vi "Beam_Max_Pos.vi"(1 "Picture Log":path, 5 "Search Step (mm)":dbl=1.0, 6 "Mode":T6, 7 "Starting Position":dbl[](array[numeric]) format="%.1f", 8 "Traverse line In":T1 {"Row Duration (mins)" format="%#.1f"; "Row No" min=0; "Trace Gas Concentration (%)" min=0.0 format="%#.2f"; "Emission Rate (l/min)" format="%#.2f"; "Tunnel Speed" format="%#.2f"; "Start X" format="%#.2f"; "Start Y" format="%#.2f"; "Start Z" format="%#.2f"; "End X" format="%#.2f"; "End Y" format="%#.2f"; "End Z" format="%#.2f"; "Averaging time (min)" min=0.0 format="%#.2f"}, 9 "Fixed Axis":T4, 10 "Beam Name":string) -> (0 "Power at Maxima":dbl, 2 "Status":T5, 3 "Beam maxima":dbl[](array[numeric]) format="%.1f", 4 "Message":string)   [LabVIEW 2010]
uses:
  Controls/User_Specific_mode.ctl
  Gen Trav/Multi_Run_Status.ctl
  Gen Trav/Route mapping/Axis.ctl
  Gen Trav/Traverse_cluster.ctl
  Gen Trav/Spacing.ctl
  Controls/Multi_run_mode.ctl
  File/Setup_Filetype.ctl
panel:
  out "Server copy Location":path
  out "vi reference":refnum<vi>
  in  "stop":bool
  out "Y":i32
  out "X":i32
  out "Array 2":dbl[](array[numeric]) format="%.4f"
  out "Measured Points":dbl[][](array[numeric]) format="%.2f"
  out "Current Value":dbl format="%.2f"
  out "Current Index":i32
  out "Array":i32[][](array[numeric])
  out "Light Power Measurement":dbl[][](graph)
  out "Found Maxima?":bool
  out "Present Position":dbl[](array[numeric])
  out "Profile":dbl[][](array[numeric]) format="%.2f"
  out "Log File":path
  # "X           Y            Z"
  # "Start"
  # "End"
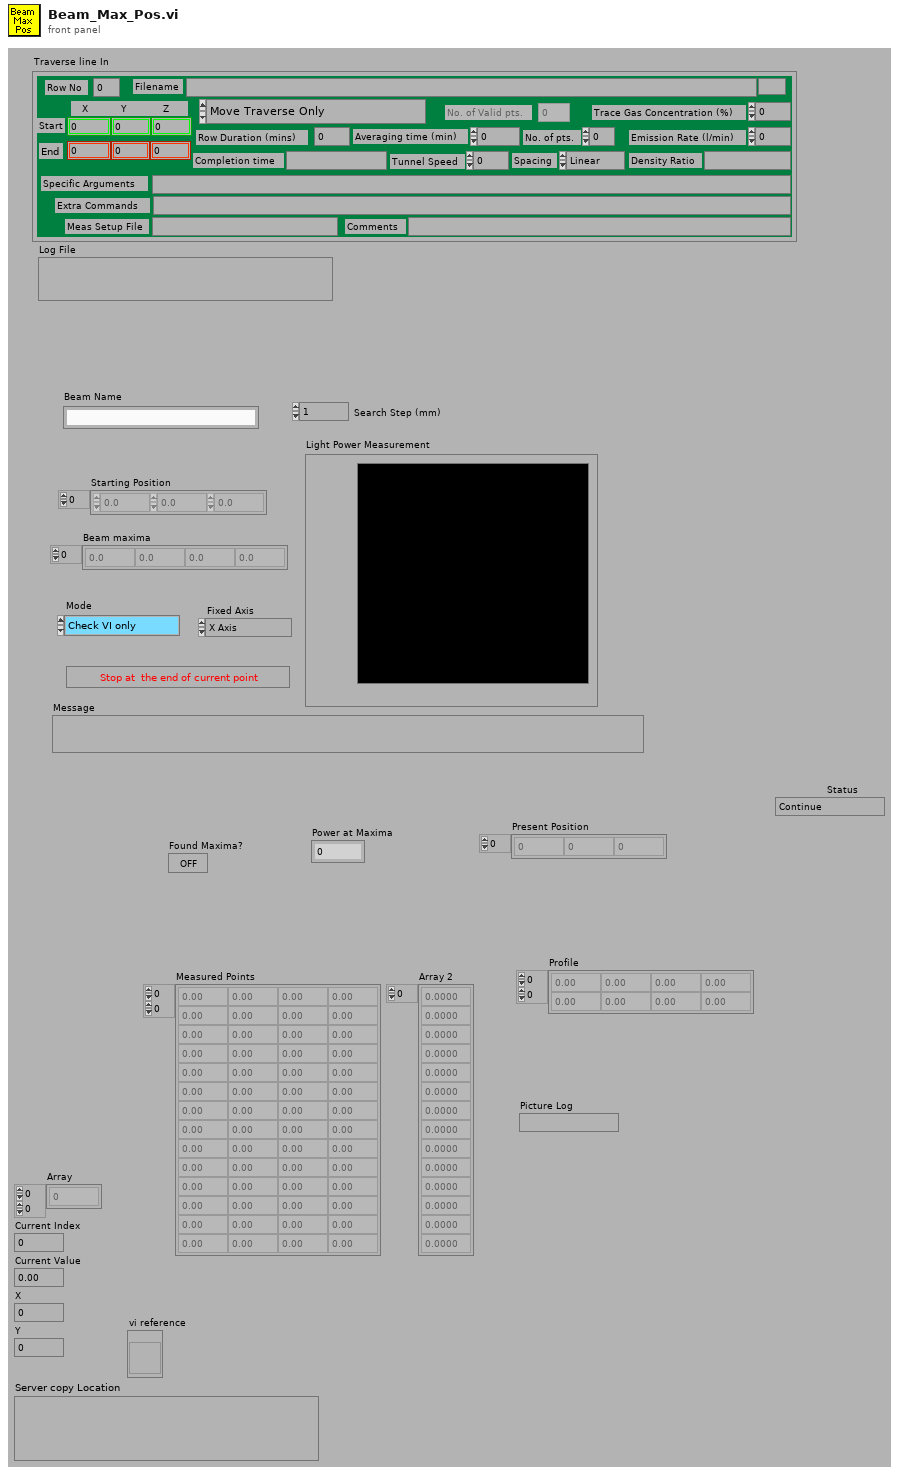
[diagram p1: front panel]
types:
  T1 = typedef "Traverse_cluster.ctl" = cluster{"Start X":dbl, "Start Y":dbl, "Start Z":dbl, "End X":dbl, "End Y":dbl, "End Z":dbl, "No. of pts.":i32, "Spacing":T2, "Filename":path, "Tunnel Speed":dbl, "Averaging time (min)":dbl, "Extra Commands":string, "Specific Arguments":string, "Emission Rate (l/min)":dbl, "Trace Gas Concentration (%)":dbl, "Density Ratio":string, "Comments":string, "Row No":i32, "Row Type Selector":T3, "Completion time":string, "Row Duration (mins)":dbl, "No. of Valid pts.":i32, "Meas Setup File":string}
  T2 = typedef "Spacing.ctl" = enum16{"Linear", "Log", "Gauss", "Specified", "N/A"}
  T3 = typedef "Multi_run_mode.ctl" = enum16{"Move Traverse Only", "Set Tunnel Speed Only", "Set Source Only", "Set Measurement Conditions", "Single Measurement", "Vertical Profile", "Lateral Profile", "Longitudinal Profile", "Explore Volume", "Multi-Axis Profile", "Auto Calibrate", "Meas Fast FID Bkgnd", "Check Beam Power", "Scanning Valve Measurement", "Run VI Named:", "Set ADAM Ch", "Wait (minutes)", "Send Message", "Synchronize With:", "Fall Back to this Row", "Turn Off Row Repeating", "Blank Row"}
  T4 = typedef "Axis.ctl" = enum16{"X Axis", "X Axis -ve", "Y Axis", "Y Axis -ve", "Z Axis", "Z Axis -ve"}
  T5 = typedef "Multi_Run_Status.ctl" = enum16{"Continue", "Jump to Next Point", "Jump to Next Row", "Jump To Fall Back", "Terminate Run"}
  T6 = typedef "User_Specific_mode.ctl" = enum16{"Check VI only", "Run VI"}
  T7 = typedef "Setup_Filetype.ctl" = enum16{"Measurement Setups", "Calibration Setups", "General", "Results File Plotter Setups", "Speed Calib Tweaks"}
  T8 = cluster{"Status":enum16{"Continue", "Jump to Next Point", "Jump to Next Row", "Jump To Fall Back", "Terminate Run"}, "Error Type":string, "Error Description":string}
  T9 = typedef "Status_Cluster.ctl" = cluster{"Status":T5, "Error Type":string, "Error Description":string}
  T10 = cluster{"second":i32, "minute":i32, "hour":i32, "day of month":i32, "month":i32, "year":i32, "day of week":i32, "day of year":i32, "is DST":i32}
  T11 = typedef "LVRectTypeDef.ctl" = cluster{"left":i16, "top":i16, "right":i16, "bottom":i16}
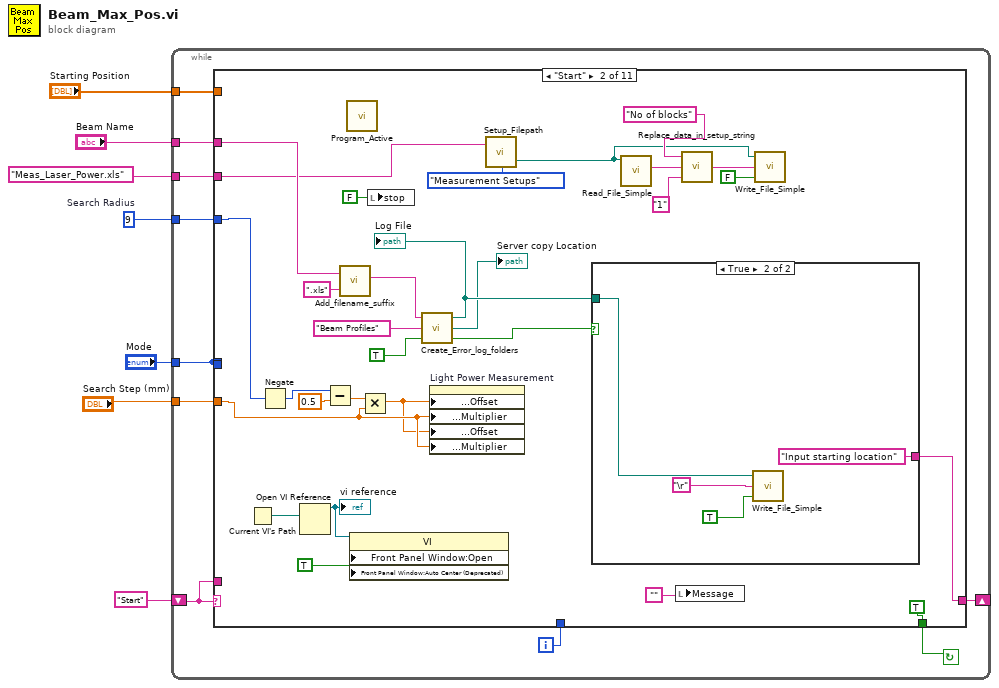
[diagram p0: block diagram]
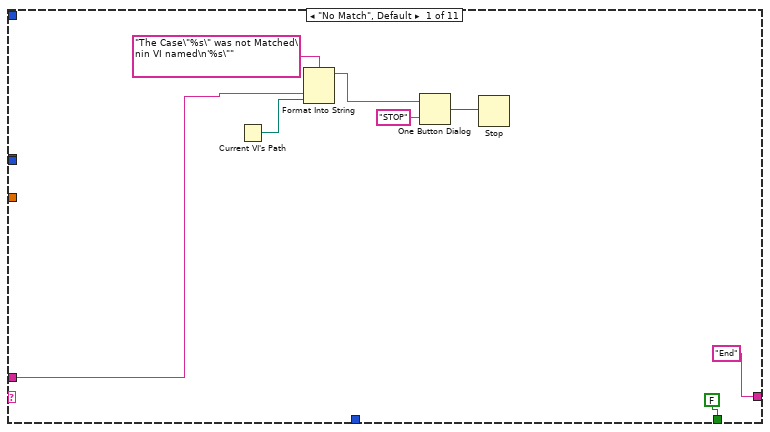
[diagram p2: hidden frame]
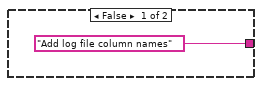
[diagram p3: hidden frame]
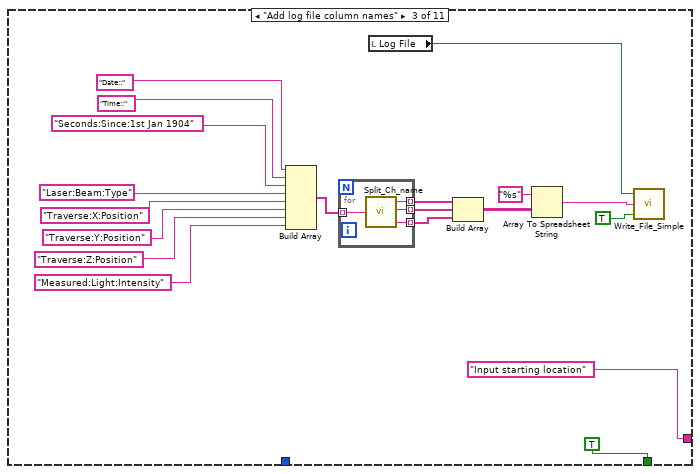
[diagram p4: hidden frame]
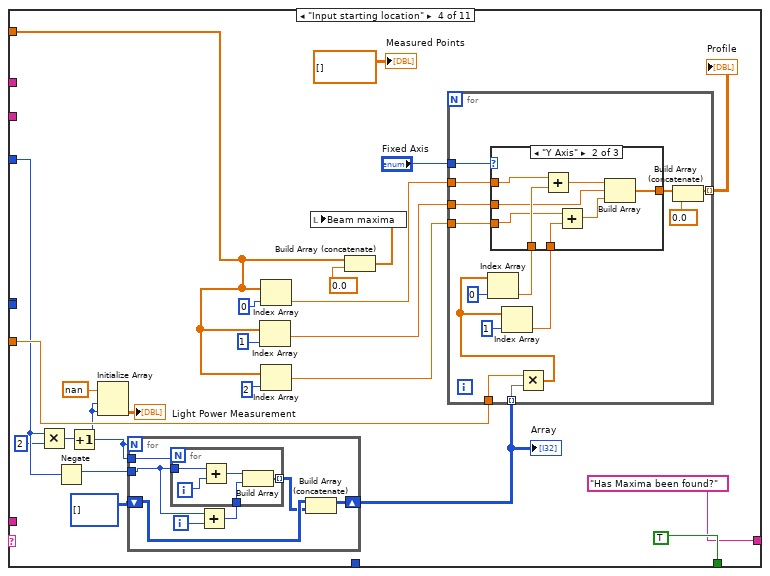
[diagram p5: hidden frame]
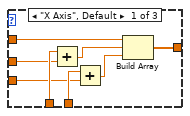
[diagram p6: hidden frame]
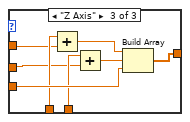
[diagram p7: hidden frame]
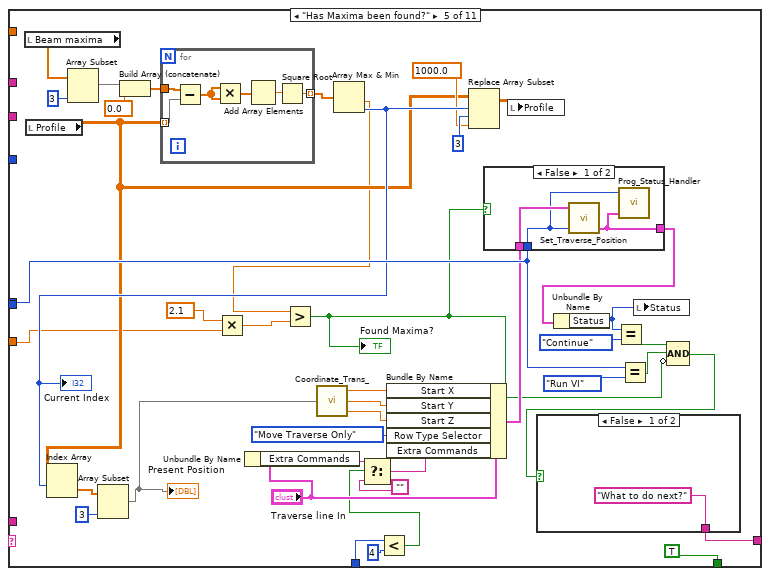
[diagram p8: hidden frame]
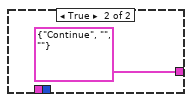
[diagram p9: hidden frame]
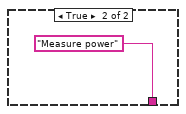
[diagram p10: hidden frame]
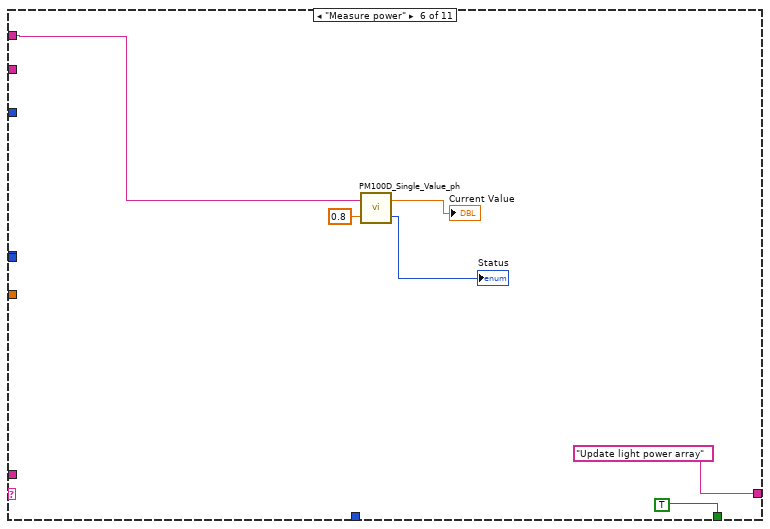
[diagram p11: hidden frame]
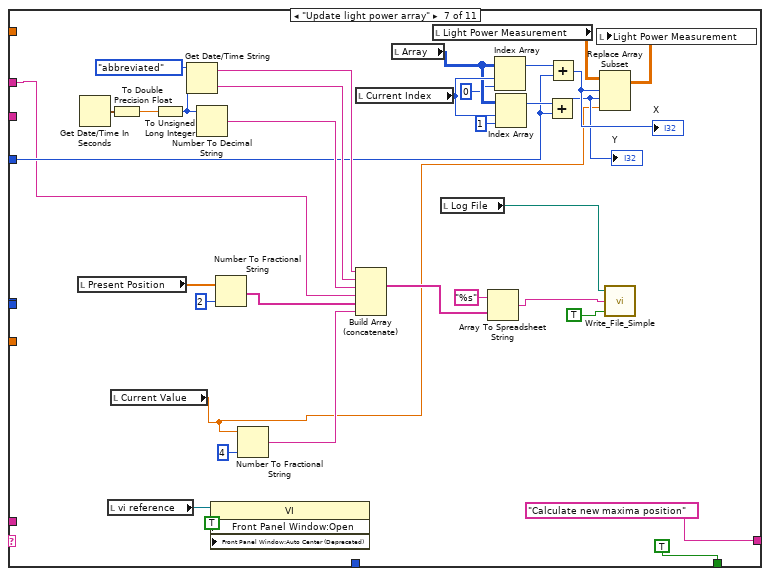
[diagram p12: hidden frame]
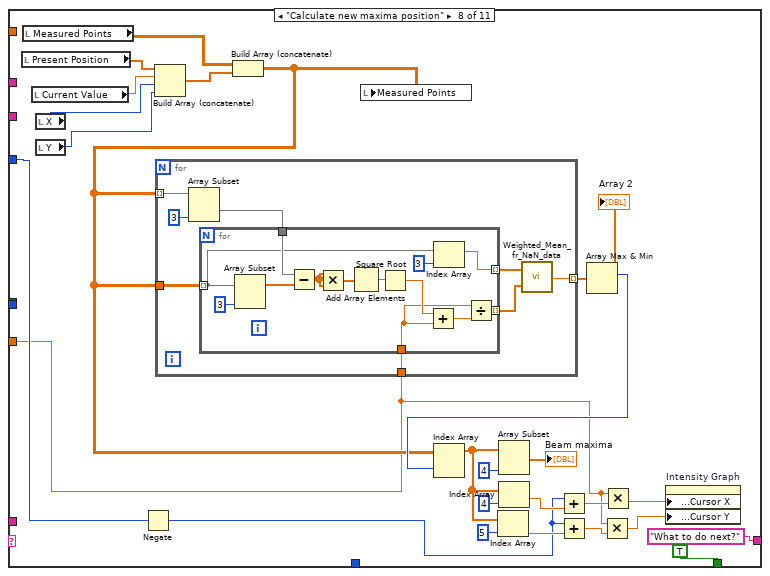
[diagram p13: hidden frame]
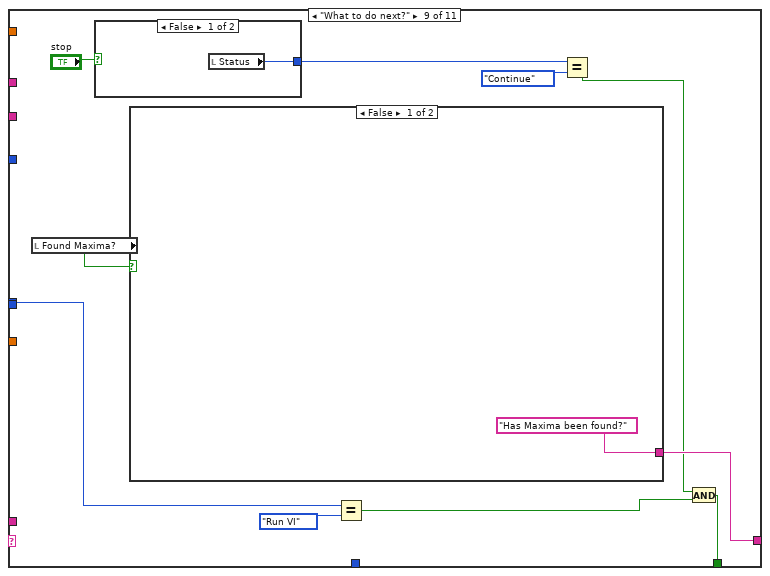
[diagram p14: hidden frame]
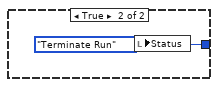
[diagram p15: hidden frame]
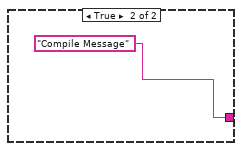
[diagram p16: hidden frame]
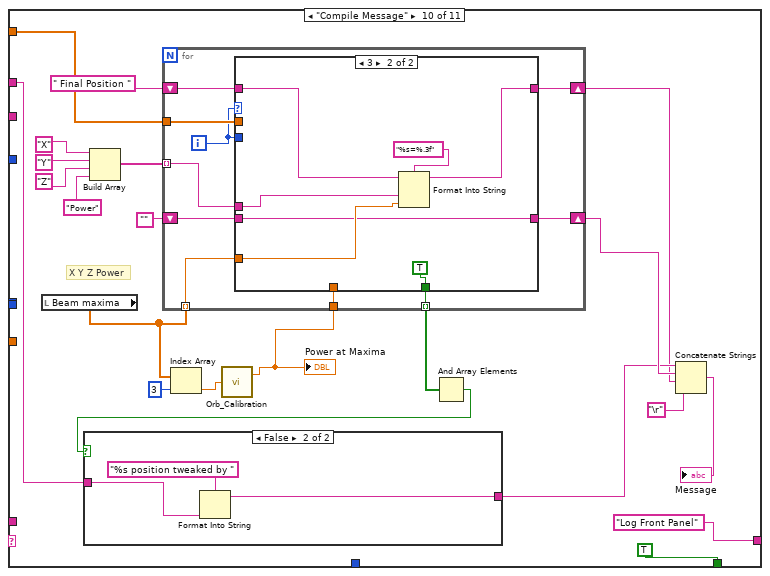
[diagram p17: hidden frame]
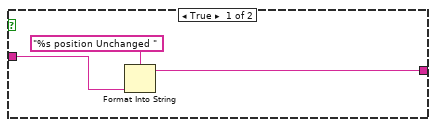
[diagram p18: hidden frame]
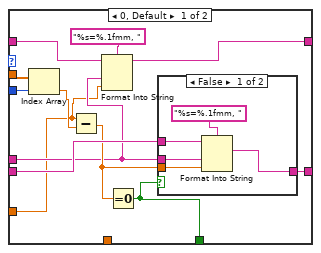
[diagram p19: hidden frame]
diagram:
  w5 = 9  # Search Radius
  n1 = while {
    tunnel: "Search Step (mm)" -> [w13]
    tunnel: "Meas_Laser_Power.xls" -> [w15]
    tunnel: "Mode" -> [w14]
    shift-left: "Start" -> [w8]
    shift-right: [w16] -> _
    tunnel: w5 -> [w12]
    tunnel: "Beam Name" -> [w11]
    tunnel: "Starting Position" -> [w10]
    i -> [w9]
    stop <- w17 continue-if-true
    n2 = case shown="\"Start\"" w8 {
      tunnel: w14 -> [_ _ _ _ w193 _ _ _ w302 _ _]
      tunnel: [FALSE TRUE TRUE TRUE TRUE TRUE TRUE TRUE w296 TRUE FALSE] -> w17
      tunnel: ["End" w44 "Input starting location" "Has Maxima been found?" w172 "Update light power array" "Calculate new maxima position" "What to do next?" w299 "Log Front Panel" "End"] -> w16
      tunnel: w15 -> [_ w27 _ _ _ _ _ _ _ _ _]
      tunnel: w14 -> [_ _ _ _ _ _ _ _ _ _ _]
      tunnel: w13 -> [_ w43 _ w99 w174 _ _ w253 _ _ _]
      tunnel: w12 -> [_ w49 _ w91 _ _ w224 w257 _ _ _]
      tunnel: w11 -> [_ w47 _ _ _ w211 w222 _ _ w322 w379]
      tunnel: w10 -> [_ _ _ w84 _ _ _ _ _ w321 _]
      tunnel: w9 -> [_ _ _ _ w157 _ _ _ _ _ _]
      tunnel: w8 -> [w20 _ _ _ _ _ _ _ _ _ _]
      frame "No Match", Default {
        n3 = Current VI's Path() -> (path=w25:path)
        n4 = Format Into String(format string="The Case\"%s\" was not Matched\nin VI named\n'%s\"" ("Format String"), w20, w25) -> (resulting string=w22:string)  [unwired: 2 in, 1 out]
        n5 = One Button Dialog(message=w22, button name ("OK")="STOP") -> (true=w24:bool)
        n6 = Stop(stop? (T)=w24) -> ()
      }
      frame "Start" {
        w37 = TRUE ("Front Panel Window:Open")
        n7 = Current VI's Path() -> (path=w38:path)
        n8 = Negate(x=w49) -> (-x=w40:i32)
        n9 = Open VI Reference(vi path=w38) -> (vi reference=w36:refnum<vi>)  [unwired: 1 in, 5 out]
        "vi reference" <- w36
        n10 = Subtract(x=w40, y=0.5) -> (x-y=w41:dbl)
        n11 = call "Add_filename_suffix.vi"("Filename"=w47, "Suffix to add"=".xls") -> ("Filename out"=w45:string)  [unwired: 3 out]
        n12 = call "Program_Active.vi"() -> ()  [unwired: 1 in]
        n13 = property class="VI"(reference=w36, "Front Panel Window:Open"=w37, "Front Panel Window:Auto Center (Deprecated)"=w37) -> ()  [unwired: 1 in, 2 out]
        n14 = Multiply(x=w41, y=w43) -> (x*y=w42:dbl)
        n15 = local write "stop"(FALSE ("stop")) -> ()
        n16 = call "Create_Error_log_folders.vi"("Per Day Log File?"=TRUE, "Log Folder"="Beam Profiles" ("Input Element"), "Log Filename"=w45) -> ("exists?"=w52:bool, "Server copy Location"=→"Server copy Location":path, "Local Log File"=w53:path)
        "Log File" <- w53
        n17 = property on="Light Power Measurement" class="IntGraph (strict)"("X Scale.Offset and Multiplier:Offset"=w42, "X Scale.Offset and Multiplier:Multiplier"=w43, "Y Scale.Offset and Multiplier:Offset"=w42, "Y Scale.Offset and Multiplier:Multiplier"=w43) -> ()  [unwired: 2 in, 2 out]
        n18 = call "Setup_Filepath.vi"("Setup File Type"=Setup_Filetype."Measurement Setups", "Filename in"=w27) -> ("Filename Out"=w26:path)  [unwired: 1 out]
        n19 = case shown="True" w52 {
          tunnel: w53 -> [_ w56]
          tunnel: ["Add log file column names" "Input starting location"] -> w44
          frame False {
          }
          frame True {
            n20 = call "Write_File_Simple.vi"("append to file? (new file:F)"=TRUE, "character string"="\r", "file path"=w56) -> ()  [unwired: 2 out]
          }
        }
        n21 = call "Read_File_Simple.vi"("Filename"=w26) -> ("string"=w29:string)  [unwired: 2 in, 7 out]
        n22 = local write "Message"("") -> ()
        n23 = call "Replace_data_in_setup_string.vi"("New data string"="1", "Input string"=w29, "Variable name"="No of blocks") -> ("Appended string"=w32:string)
        n24 = call "Write_File_Simple.vi"("append to file? (new file:F)"=FALSE, "character string"=w32, "file path"=w26) -> ()  [unwired: 2 out]
      }
      frame "Add log file column names" {
        n25 = Build Array("Date::", "Time::", "Seconds:Since:1st Jan 1904", "Laser:Beam:Type", "Traverse:X:Position", "Traverse:Y:Position", "Traverse:Z:Position", "Measured:Light:Intensity") -> (w72:string[])
        n26 = for {
          tunnel: w72 -> [w82] mode=indexing
          tunnel: [w81] -> w73 mode=indexing
          tunnel: [w80] -> w74 mode=indexing
          tunnel: [w79] -> w75 mode=indexing
          n27 = call "Split_Ch_name.vi"("Ch name"=w82) -> ("Top level"=w81:string, "Middle"=w80:string, "Low level"=w79:string)
        }
        n28 = local read "Log File"() -> (w60:path)
        n29 = Build Array(w73, w74, w75) -> (w70:string[][])
        n30 = Array To Spreadsheet String(array=w70, 3:"%s" ("format string")) -> (spreadsheet string=w61:string)  [unwired: 1 out]
        n31 = call "Write_File_Simple.vi"("append to file? (new file:F)"=TRUE, "character string"=w61, "file path"=w60) -> ()  [unwired: 2 out]
      }
      frame "Input starting location" {
        n32 = Multiply(x=w91, y=2) -> (x*y=w89:i32)
        n33 = Negate(x=w91) -> (-x=w92:i32)
        n34 = Increment(x=w89) -> (x+1=w88:i32)
        n35 = Initialize Array(nan, w88, w88) -> (→"Light Power Measurement":dbl[][])
        n36 = for {
          N: w88 -> [_]
          tunnel: w88 -> [w113]
          tunnel: w92 -> [w111]
          shift-right: [w107] -> w97
          shift-left: i32[][] [] -> [w109]
          i -> [w112]
          n37 = Add(x=w111, y=w112) -> (x+y=w110:i32)
          n38 = for {
            N: w113 -> [_]
            tunnel: w111 -> [w117]
            tunnel: w110 -> [w115]
            tunnel: [w114] -> w108 mode=indexing
            i -> [w118]
            n39 = Add(x=w117, y=w118) -> (x+y=w116:i32)
            n40 = Build Array(w116, w115) -> (w114:i32[])
          }
          n41 = Build Array (concatenate)(w109, w108) -> (w107:i32[][])
        }
        "Array" <- w97
        n42 = Index Array(array=w84, index=1 ("Index")) -> (element=w103:dbl)
        n43 = Index Array(array=w84, index=0 ("Index")) -> (element=w104:dbl)
        n44 = Index Array(array=w84, index=2 ("Index")) -> (element=w102:dbl)
        n45 = Build Array (concatenate)(w84, 0.0 ("Numeric")) -> (w100:dbl[])
        n46 = local write "Beam maxima"(w100) -> ()
        n47 = for {
          tunnel: w99 -> [w132]
          tunnel: w97 -> [w131] mode=indexing
          tunnel: "Fixed Axis" -> [w130]
          tunnel: w104 -> [w126]
          tunnel: w103 -> [w123]
          tunnel: w102 -> [w122]
          tunnel: [w120] -> w105 mode=indexing
          n48 = Multiply(x=w132, y=w131) -> (x*y=w127:dbl[])
          n49 = Index Array(array=w127, index=0 ("Index")) -> (element=w125:dbl)
          n50 = Index Array(array=w127, index=1 ("Index")) -> (element=w124:dbl)
          n51 = case shown="\"Y Axis\"" w130 {
            tunnel: w126 -> [w140 w147 w151]
            tunnel: w125 -> [w139 w145 w154]
            tunnel: w124 -> [w138 w144 w153]
            tunnel: w123 -> [w137 w141 w152]
            tunnel: w122 -> [w136 w143 w155]
            tunnel: [w133 w148 w156] -> w121
            frame "X Axis", Default {
              n52 = Add(x=w139, y=w137) -> (x+y=w135:dbl)
              n53 = Add(x=w138, y=w136) -> (x+y=w134:dbl)
              n54 = Build Array(w140, w135, w134) -> (w133:dbl[])
            }
            frame "Y Axis" {
              n55 = Add(x=w147, y=w145) -> (x+y=w146:dbl)
              n56 = Add(x=w143, y=w144) -> (x+y=w142:dbl)
              n57 = Build Array(w146, w141, w142) -> (w148:dbl[])
            }
            frame "Z Axis" {
              n58 = Add(x=w154, y=w151) -> (x+y=w150:dbl)
              n59 = Add(x=w153, y=w152) -> (x+y=w149:dbl)
              n60 = Build Array(w150, w149, w155) -> (w156:dbl[])
            }
          }
          n61 = Build Array (concatenate)(w121, 0.0 ("Input Element")) -> (w120:dbl[])
        }
        "Profile" <- w105
        "Measured Points" <- dbl[][] [] ("Measured Points")
      }
      frame "Has Maxima been found?" {
        n62 = local read "Beam maxima"() -> (w190:dbl[])
        n63 = local read "Profile"() -> (w180:dbl[][])
        n64 = Array Subset(array=w190, length=3 ("Array Length")) -> (w187:dbl[])  [unwired: 1 in]
        n65 = Build Array (concatenate)(w187, 0.0 ("Input Element")) -> (w186:dbl[])
        n66 = for {
          tunnel: w180 -> [w209] mode=indexing
          tunnel: w186 -> [w208]
          tunnel: [w204] -> w188 mode=indexing
          n67 = Subtract(x=w208, y=w209) -> (x-y=w206:dbl[])
          n68 = Multiply(x=w206, y=w206) -> (x*y=w205:dbl[])
          n69 = Add Array Elements(numeric array=w205) -> (sum=w207:dbl)
          n70 = Square Root(x=w207) -> (sqrt(x)=w204:dbl)
        }
        n71 = Multiply(x=2.1, y=w174) -> (x*y=w177:dbl)
        n72 = Unbundle By Name("Traverse line In") -> ("Extra Commands"=w169:string)
        n73 = Array Max & Min(array=w188) -> (min value=w178:dbl, min index (indices)=w184:i32)  [unwired: 2 out]
        "Current Index" <- w184
        n74 = Index Array(array=w180, index (row)=w184) -> (element=w160:dbl[])  [unwired: 1 in]
        n75 = Array Subset(array=w160, length=3) -> (w159:dbl[])  [unwired: 1 in]
        "Present Position" <- w159
        n76 = Greater?(x=w178, y=w177) -> (0:w164:bool)
        "Found Maxima?" <- w164
        n77 = call "Coordinate_Trans_.vi"("Input Position"=w159) -> ("X"=w161:dbl, "Y"=w162:dbl, "Z"=w163:dbl)
        n78 = Less?(x=w157, y=4) -> (x < y?=w167:bool)
        n79 = Select(t=w169, s=w167, f="") -> (s? t:f=w165:string)
        n80 = Bundle By Name(cluster="Traverse line In", "Start X"=w161, "Start Y"=w162, "Start Z"=w163, "Row Type Selector"=Multi_run_mode."Move Traverse Only", "Extra Commands"=w165) -> (w173:T1)
        n81 = Replace Array Subset(array=w180, new element=1000.0 ("Element Data"), index (row)=w184, index (col)=3 ("Index")) -> (w181:dbl[][])
        n82 = case shown="False" w164 {
          tunnel: [w199 T8 {"Status"=enum."Continue", "Error Type"="", "Error Description"=""} ("Status Cluster")] -> w195
          tunnel: w193 -> [w198 _]
          tunnel: w173 -> [w200 _]
          frame False {
            n83 = call "Set_Traverse_Position.vi"("Simulate/Run"=w198, "Traverse line"=w200) -> ("Status Cluster"=w199:T9)  [unwired: 1 in, 2 out]
            n84 = call "Prog_Status_Handler.vi"("Status Cluster"=w199, "Simulate/Run"=w198) -> ()  [unwired: 2 out]
          }
          frame True {
          }
        }
        n85 = local write "Profile"(w181) -> ()
        n86 = Unbundle By Name(w195) -> ("Status"=w191:T5)
        n87 = Equal?(x=w191, y=Multi_Run_Status."Continue" ("Status")) -> (x = y?=w176:bool)
        n88 = Equal?(x=w193, y=User_Specific_mode."Run VI" ("Mode")) -> (x = y?=w175:bool)
        n89 = local write "Status"(w191) -> ()
        n90 = Compound Arithmetic op=AND(w176, w175, invert w164) -> (w171:bool)
        n91 = case shown="False" w171 {
          tunnel: ["What to do next?" "Measure power"] -> w172
          frame False {
          }
          frame True {
          }
        }
      }
      frame "Measure power" {
        n92 = call "PM100D_Single_Value_ph.vi"("Averaging Period (s)"=0.8, "Beam Name"=w211) -> ("Status"=→"Status":T5, "Light Power mW"=→"Current Value":dbl)
      }
      frame "Update light power array" {
        w220 = TRUE ("Front Panel Window:Open")
        n93 = local read "Present Position"() -> (w236:dbl[])
        n94 = Get Date/Time In Seconds() -> (seconds since 1Jan1904=w225:timestamp)
        n95 = local read "vi reference"() -> (w221:refnum<vi>)
        n96 = local read "Current Value"() -> (w216:dbl)
        n97 = To Double Precision Float(number=w225) -> (double precision float=w246:dbl)
        n98 = To Unsigned Long Integer(number=w246) -> (unsigned 32bit integer=w245:u32)
        n99 = Get Date/Time String(date format (0)=enum16{"short", "long", "abbreviated"}."abbreviated", seconds (now)=w245) -> (date string=w244:string, time string=w243:string)  [unwired: 1 out]
        n100 = Number To Decimal String(number=w245) -> (decimal integer string=w242:string)  [unwired: 1 out]
        n101 = property class="VI"(reference=w221, "Front Panel Window:Open"=w220, "Front Panel Window:Auto Center (Deprecated)"=w220) -> ()  [unwired: 1 in, 2 out]
        n102 = Number To Fractional String(number=w236, precision (6)=i16 2) -> (F-format string=w237:string[])  [unwired: 2 out]
        n103 = Number To Fractional String(number=w216, precision (6)=i16 4) -> (F-format string=w238:string)  [unwired: 2 out]
        n104 = local read "Current Index"() -> (w235:i32)
        n105 = Build Array (concatenate)(w244, w243, w242, w222, w237, w238) -> (w241:string[])
        n106 = local read "Array"() -> (w234:i32[][])
        n107 = local read "Light Power Measurement"() -> (w231:dbl[][])
        n108 = local read "Log File"() -> (w217:path)
        n109 = Array To Spreadsheet String(array=w241, 3:"%s" ("format string")) -> (spreadsheet string=w218:string)  [unwired: 1 out]
        n110 = Index Array(array=w234, index (row)=w235, index (col)=0 ("Index")) -> (element=w228:i32)
        n111 = Index Array(array=w234, index (row)=w235, index (col)=1 ("Index")) -> (element=w229:i32)
        n112 = Add(x=w229, y=w224) -> (x+y=w226:i32)
        "Y" <- w226
        n113 = Add(x=w228, y=w224) -> (x+y=w227:i32)
        "X" <- w227
        n114 = Replace Array Subset(array=w231, new element=w216, index (row)=w227, index (col)=w226) -> (w230:dbl[][])
        n115 = local write "Light Power Measurement"(w230) -> ()
        n116 = call "Write_File_Simple.vi"("append to file? (new file:F)"=TRUE, "character string"=w218, "file path"=w217) -> ()  [unwired: 2 out]
      }
      frame "Calculate new maxima position" {
        n117 = local read "Present Position"() -> (w272:dbl[])
        n118 = local read "Measured Points"() -> (w273:dbl[][])
        n119 = local read "Current Value"() -> (w271:dbl)
        n120 = local read "X"() -> (w266:i32)
        n121 = local read "Y"() -> (w265:i32)
        n122 = Negate(x=w257) -> (-x=w255:i32)
        n123 = Build Array (concatenate)(w272, w271, w266, w265) -> (w270:dbl[])
        n124 = Build Array (concatenate)(w273, w270) -> (w267:dbl[][])
        n125 = for {
          tunnel: w267 -> [w282] mode=indexing
          tunnel: w267 -> [w280]
          tunnel: w253 -> [w278]
          tunnel: [w275] -> w269 mode=indexing
          n126 = Array Subset(array=w282, length=3 ("Array Length")) -> (w279:dbl[])  [unwired: 1 in]
          n127 = for {
            tunnel: w280 -> [w289] mode=indexing
            tunnel: w279 -> [w294]
            tunnel: w278 -> [w284]
            tunnel: [w286] -> w276 mode=indexing
            tunnel: [w283] -> w277 mode=indexing
            n128 = Array Subset(array=w289, length=3 ("Array Length")) -> (w293:dbl[])  [unwired: 1 in]
            n129 = Subtract(x=w294, y=w293) -> (x-y=w290:dbl[])
            n130 = Multiply(x=w290, y=w290) -> (x*y=w291:dbl[])
            n131 = Add Array Elements(numeric array=w291) -> (sum=w292:dbl)
            n132 = Square Root(x=w292) -> (sqrt(x)=w287:dbl)
            n133 = Add(x=w287, y=w284) -> (x+y=w285:dbl)
            n134 = Index Array(array=w289, index=3 ("Index")) -> (element=w283:dbl)
            n135 = Divide(x=w284, y=w285) -> (x/y=w286:dbl)
          }
          n136 = call "Weighted_Mean_fr_NaN_data.vi"("Weighting"=w276, "Data"=w277) -> ("Mean value"=w275:dbl)
        }
        "Array 2" <- w269
        n137 = local write "Measured Points"(w267) -> ()
        n138 = Array Max & Min(array=w269) -> (max index (indices)=w268:i32)  [unwired: 3 out]
        n139 = Index Array(array=w267, index (row)=w268) -> (element=w260:dbl[])  [unwired: 1 in]
        n140 = Index Array(array=w260, index=5 ("Index")) -> (element=w258:dbl)
        n141 = Array Subset(array=w260, length=4 ("Array Length")) -> (→"Beam maxima":dbl[])  [unwired: 1 in]
        n142 = Index Array(array=w260, index=4 ("Index")) -> (element=w259:dbl)
        n143 = Add(x=w255, y=w259) -> (x+y=w254:dbl)
        n144 = Add(x=w255, y=w258) -> (x+y=w252:dbl)
        n145 = Multiply(x=w253, y=w252) -> (x*y=w251:dbl)
        n146 = Multiply(x=w253, y=w254) -> (x*y=w250:dbl)
        n147 = property on="Intensity Graph" class="IntGraph (strict)"("Cursor.Cursor Position:Cursor X"=w250, "Cursor.Cursor Position:Cursor Y"=w251) -> ()  [unwired: 2 in, 2 out]
      }
      frame "What to do next?" {
        n148 = local read "Found Maxima?"() -> (w304:bool)
        n149 = case shown="False" "stop" {
          tunnel: [w306 w307] -> w300
          frame False {
            n150 = local read "Status"() -> (w306:T5)
          }
          frame True {
            w307 = Multi_Run_Status."Terminate Run" ("Status")
            n151 = local write "Status"(w307) -> ()
          }
        }
        n152 = case shown="False" w304 {
          tunnel: ["Has Maxima been found?" "Compile Message"] -> w299
          frame False {
          }
          frame True {
          }
        }
        n153 = Equal?(x=w302, y=User_Specific_mode."Run VI" ("Mode")) -> (x = y?=w298:bool)
        n154 = Equal?(x=w300, y=Multi_Run_Status."Continue" ("Status")) -> (x = y?=w297:bool)
        n155 = And(x=w297, y=w298) -> (x .and. y?=w296:bool)
      }
      frame "Compile Message" {
        # "X Y Z Power"
        n156 = local read "Beam maxima"() -> (w320:dbl[])
        n157 = Build Array("X", "Y", "Z", "Power" ("Input Element")) -> (w327:string[])
        n158 = Index Array(array=w320, index=3) -> (element=w318:dbl)
        n159 = call "Orb_Calibration.vi"("Voltage"=w318) -> ("Normalised Voltage"=w316:dbl)  [unwired: 1 out]
        "Power at Maxima" <- w316
        n160 = for {
          tunnel: w320 -> [w347] mode=indexing
          shift-right: [w345] -> w326
          shift-left: "" -> [w346]
          tunnel: w327 -> [w344] mode=indexing
          tunnel: [w343] -> w323 mode=indexing
          tunnel: w321 -> [w342]
          tunnel: w316 -> [w340]
          shift-right: [w338] -> w312
          shift-left: " Final Position " -> [w339]
          i -> [w341]
          n161 = case shown="3" w341 {
            tunnel: w347 -> [w349 w370]
            tunnel: w346 -> [w359 w366]
            tunnel: [w358 w366] -> w345
            tunnel: w344 -> [w350 w372]
            tunnel: [w356 TRUE] -> w343
            tunnel: w342 -> [w355 _]
            tunnel: w341 -> [w354 _]
            tunnel: w340 -> [_ _]
            tunnel: w339 -> [w351 w368]
            tunnel: [w348 w367] -> w338
            frame 0, Default {
              n162 = Index Array(array=w355, index=w354) -> (element=w353:dbl)
              n163 = Subtract(x=w349, y=w353) -> (x-y=w357:dbl)
              n164 = Format Into String(format string="%s=%.1fmm, " ("Format String"), initial string=w351, w350, w349) -> (resulting string=w348:string)  [unwired: 1 in, 1 out]
              n165 = Equal To 0?(x=w357) -> (x = 0?=w356:bool)
              n166 = case shown="False" w356 {
                tunnel: w359 -> [w364 w365]
                tunnel: [w363 w365] -> w358
                tunnel: w350 -> [w362 _]
                tunnel: w357 -> [w360 _]
                frame False {
                  n167 = Format Into String(format string="%s=%.1fmm, " ("Format String"), initial string=w364, w362, w360) -> (resulting string=w363:string)  [unwired: 1 in, 1 out]
                }
                frame True {
                }
              }
            }
            frame 3 {
              n168 = Format Into String(format string="%s=%.3f" ("Format String"), initial string=w368, w372, w370) -> (resulting string=w367:string)  [unwired: 1 in, 1 out]
            }
          }
        }
        n169 = And Array Elements(Boolean array=w323) -> (logical AND=w315:bool)
        n170 = case shown="False" w315 {
          tunnel: [w333 w336] -> w325
          tunnel: w322 -> [w332 w335]
          frame True {
            n171 = Format Into String(format string="%s position Unchanged " ("Format String"), w332) -> (resulting string=w333:string)  [unwired: 2 in, 1 out]
          }
          frame False {
            n172 = Format Into String(format string="%s position tweaked by " ("Format String"), w335) -> (resulting string=w336:string)  [unwired: 2 in, 1 out]
          }
        }
        n173 = Concatenate Strings(w325, w326, w312, "\r") -> (→"Message":string)
      }
      frame "Log Front Panel" {
        w386 = 8 ("image depth")
        n174 = local read "Server copy Location"() -> (w373:path)
        n175 = Empty String/Path?(string/path="Picture Log") -> (empty?=w384:bool)
        n176 = local read "vi reference"() -> (w377:refnum<vi>)
        n177 = local read "Log File"() -> (w374:path)
        n178 = case shown="True" w384 {
          tunnel: [w395 w398] -> w383
          tunnel: "Picture Log" -> [w395 _]
          frame False {
          }
          frame True {
            n179 = Get Date/Time In Seconds() -> (seconds since 1Jan1904=w396:timestamp)
            n180 = call <vilib>:"LV70TimeStampToDateRec.vi"("time stamp"=w396) -> ("date time rec"=w401:T10)
            n181 = Unbundle By Name(w401) -> ("day of month"=w404:i32, "hour"=w403:i32, "minute"=w402:i32)
            n182 = call "Create_Error_log_folders.vi"("Log Folder"="Beam_Max_Pos" ("name or relative path"), "Log Filename"="test") -> ("Server copy Location"=w397:path)  [unwired: 1 in, 2 out]
            n183 = Strip Path(path=w397) -> (stripped path=w400:path)  [unwired: 1 out]
            n184 = Format Into String(format string="Day%02d_Time%02d-%02d", w404, w403, w402) -> (resulting string=w399:string)  [unwired: 2 in, 1 out]
            n185 = Build Path(base path=w400, name or relative path=w399) -> (appended path=w398:path)
          }
        }
        n186 = Close Reference(reference=w377) -> ()  [unwired: 1 in, 1 out]
        n187 = call "Updated_File_Copy.vi"("Target Path"=w373, "Source Path"=w374) -> ()  [unwired: 2 out]
        n188 = Current VI's Path() -> (path=w394:path)
        n189 = Open VI Reference(vi path=w394) -> (vi reference=w393:refnum<vi>, error out=w392:errorcluster)  [unwired: 1 in, 4 out]
        n190 = invoke class="VI" method="FP.Old Get Image"(reference=w393, error in=w392, "visible area only"=TRUE, "image depth"=w386) -> (error out=w390:errorcluster, "image"=w389:u8[], "colors"=w387:u32[], "bounds"=w388:T11)  [unwired: 4 in, 4 out]
        n191 = Concatenate Strings(w379, ".png" ("string")) -> (w380:string)
        n192 = Build Path(base path=w383, name or relative path=w380) -> (appended path=w376:path)
        n193 = call "Create_directory_path.vi"("Path name"=w376) -> ("Path name Out"=w375:path)
        n194 = call <vilib>:"Write PNG File(6_1).vi"("color table"=w387, "depth"=w386, "error in (no error)"=w390, "flattened image data"=w389, "rect"=w388, "path to PNG file"=w375) -> ()  [unwired: 6 out]
      }
    }
  }
